vi "堆栈数据结构.vi"() -> ()   [LabVIEW 2011]
uses:
  Control 1.ctl
panel:
  out "栈长度":i32
  in  "Variant 2":variant
  out "Variant":variant
  in  "Action":T1
  out "error constant 2":errorcluster
  in  "error constant":errorcluster
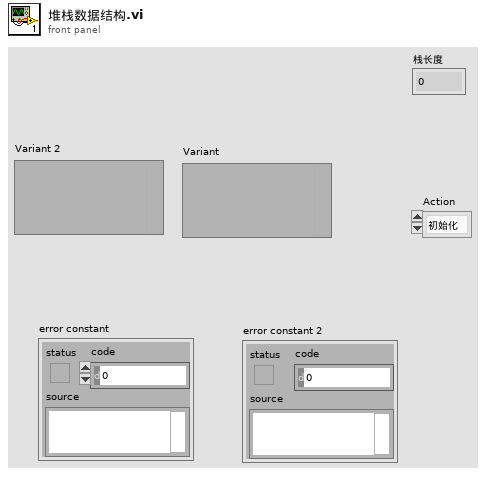
[diagram p1: front panel]
types:
  T1 = typedef "Control 1.ctl" = enum16{"初始化", "进栈", "出栈", "栈的长度"}
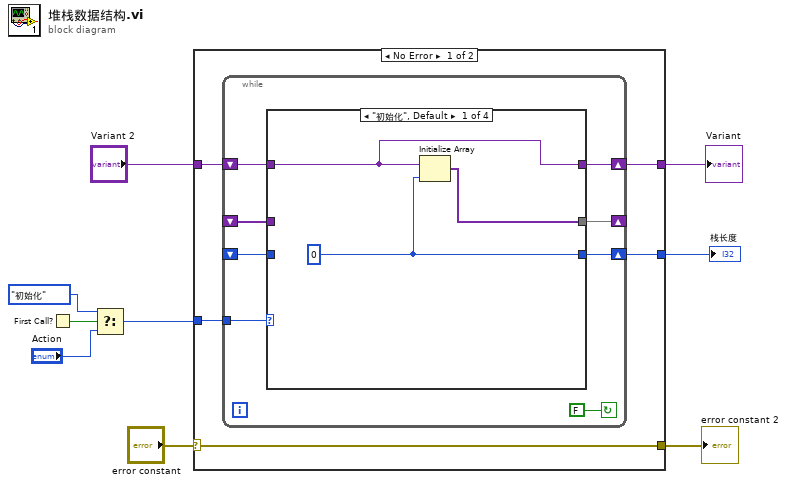
[diagram p0: block diagram]
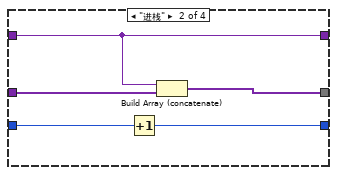
[diagram p2: hidden frame]
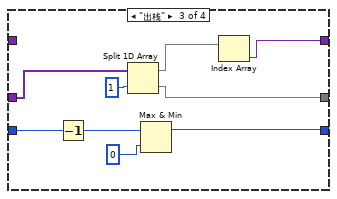
[diagram p3: hidden frame]
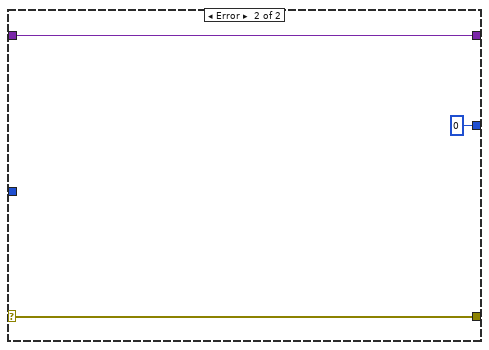
[diagram p5: hidden frame]
diagram:
  n1 = First Call?() -> (First Call?: T/F=w7:bool)
  n2 = Select(t=Control_1."初始化", s=w7, f="Action") -> (s? t:f=w4:T1)
  n3 = case shown="No Error" "error constant" {
    selector: "error constant" -> [w14 w45]
    tunnel: [w14 w45] -> w8
    tunnel: w4 -> [w13 _]
    tunnel: "Variant 2" -> [w12 w44]
    tunnel: [w11 w44] -> w2
    tunnel: [w10 0] -> w1
    frame No Error {
      n4 = while {
        tunnel: w13 -> [w22]
        shift-right: [w20] -> w11
        shift-left: w12 -> [w21]
        shift-right: [w17] -> _
        shift-left: _ -> [w16]
        shift-right: [w19] -> w10
        shift-left: _ -> [w15]
        stop <- FALSE continue-if-true
        n5 = case shown="\"初始化\", Default" w22 {
          tunnel: w21 -> [w24 w30 _ w42]
          tunnel: [w24 w30 w31 w42] -> w20
          tunnel: [w25 w26 w37 w40] -> w19
          tunnel: [w23 w29 w32 w41] -> w17
          tunnel: w16 -> [_ w28 w35 w41]
          tunnel: w15 -> [_ w27 w39 w40]
          frame "初始化", Default {
            w25 = 0
            n6 = Initialize Array(w24, w25) -> (w23:variant[])
          }
          frame "进栈" {
            n7 = Increment(x=w27) -> (x+1=w26:i32)
            n8 = Build Array (concatenate)(w30, w28) -> (w29:variant[])
          }
          frame "出栈" {
            n9 = Decrement(x=w39) -> (x-1=w36:i32)
            n10 = Split 1D Array(array=w35, index=1) -> (first subarray=w33:variant[], second subarray=w32:variant[])
            n11 = Max & Min(x=w36, y=0) -> (max(x,y)=w37:i32)  [unwired: 1 out]
            n12 = Index Array(array=w33) -> (element=w31:variant)  [unwired: 1 in]
          }
          frame "栈的长度" {
          }
        }
      }
    }
    frame Error {
    }
  }
  "error constant 2" <- w8
  "Variant" <- w2
  "栈长度" <- w1
